vi "Front Panel.vi"(11 "GUI In":refnum<class "CRD Derived.lvclass">) -> ()   [LabVIEW 2015, in "CRD Derived.lvclass"]
uses:
  CRD Derived.lvclass
  Reusable/Xctls/Buffer/2D Control/2D Buffer Display.xctl
  Reusable/GUI/GUI.lvclass/GUI.ctl
  Reusable/Observer/Observer.lvclass/Observer.ctl
  CRDS/Data/cCRDS Data.lvclass
  Reusable/CRDS/Data/Cell/CRDS Cell Data.lvclass/CRDS Cell Data.ctl
  Reusable/CRDS/Data/Cell/Read extParam.vi
  Reusable/GUI/Accessors/Read RegEvent.vi
  Reusable/Observer/Read Data Queue.vi
  Reusable/CRDS/Data/Main/Read CellData.vi
  Reusable/Data/Read measTime.vi
  Reusable/Data/Data.lvclass
  Reusable/CRDS/Data/Cell/CRDS Cell Data.lvclass
panel:
  out "extWvfm":cluster{"data_out":sgl[][], "time":timestamp}(xcontrol)
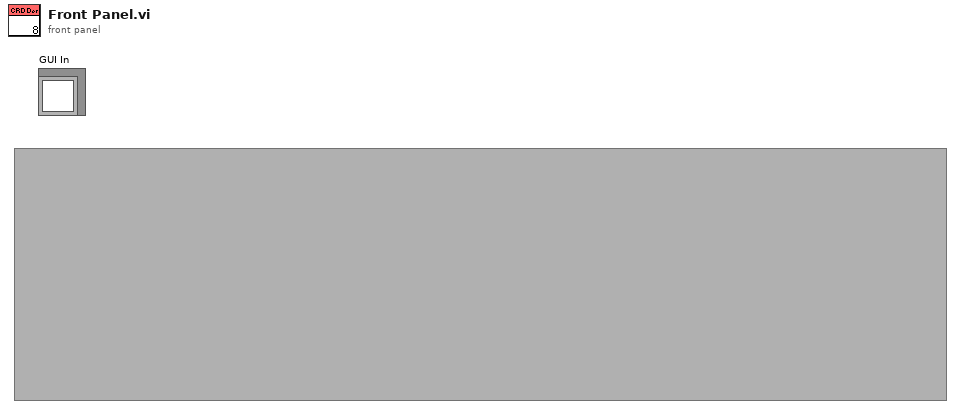
[diagram p1: front panel]
types:
  T1 = cluster{"Name":string, "Line Width":u8, "Line Style":u8, "Color":u32}[]
  T2 = typedef "extparam.ctl" = cluster{"Tau":sgl, "Tau0cor":sgl, "ext":sgl, "extCorr":sgl, "stdevTau":sgl, "eTau":sgl, "taucorr":sgl, "Tau0":sgl, "max":sgl}
  T3 = cluster{"Data Access:extParam":sgl[][], "Time":timestamp}
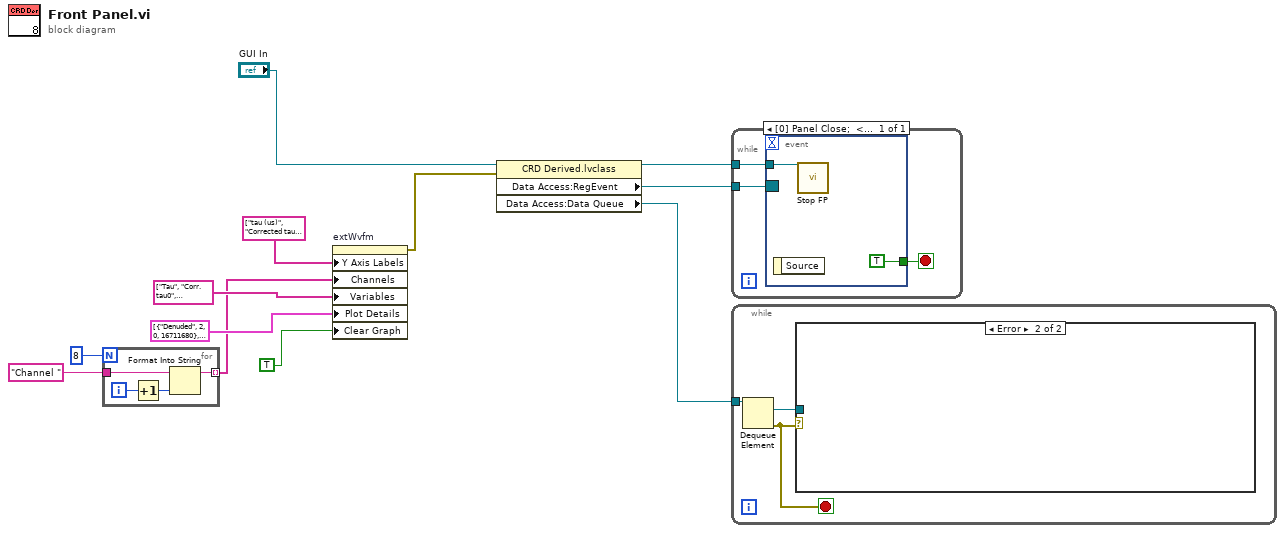
[diagram p0: block diagram]
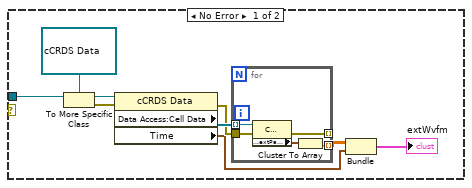
[diagram p2: hidden frame]
diagram:
  n1 = for {
    N: 8 -> [_]
    tunnel: "Channel " -> [w14]
    tunnel: [w13] -> w5 mode=indexing
    i -> [w16]
    n2 = Increment(x=w16) -> (x+1=w15:i32)
    n3 = Format Into String(initial string=w14, w15) -> (resulting string=w13:string)  [unwired: 2 in, 1 out]
  }
  n4 = property on="extWvfm" class="2D Buffer Display (strict)"("Y Axis Labels"=string[] ["tau (us)", "Corrected tau0 (us)", "Extinction (Mm-1)", "Corrected Extinction (Mm-1)", "Std. Dev. in tau (us)", "Error in tau", "Corrected tau (us)", "tau0 (us)", "Max Amplitude"], "Channels"=w5, "Variables"=string[] ["Tau", "Corr.  tau0", "Extinction", "Corrected Extinction", "Std. Dev. in tau", "Error in tau", "Corrected tau", "tau0", "Max Amplitude"], "Plot Details"=T1 [{"Name"="Denuded", "Line Width"=2, "Line Style"=0, "Color"=16711680}, {"Name"="Denuded", "Line Width"=2, "Line Style"=1, "Color"=16860}, {"Name"="Gas", "Line Width"=2, "Line Style"=0, "Color"=33023}, {"Name"="Dry", "Line Width"=2, "Line Style"=0, "Color"=16512}, {"Name"="Dry", "Line Width"=2, "Line Style"=0, "Color"=8388672}, {"Name"="Dry", "Line Width"=2, "Line Style"=1, "Color"=6618880}, {"Name"="Med RH", "Line Width"=2, "Line Style"=1, "Color"=1985280}, {"Name"="High RH", "Line Width"=2, "Line Style"=1, "Color"=32832}], "Clear Graph"=TRUE) -> (error out=w2:errorcluster)  [unwired: 2 in, 1 out]
  n5 = property class="CRD Derived.lvclass"(reference="GUI In", error in=w2) -> (reference out=w1:refnum<class "CRD Derived.lvclass">, "Data Access:RegEvent"=w12:refnum<event-registration>, "Data Access:Data Queue"=w11:refnum<queue>)  [unwired: 1 out]
  n6 = while {
    tunnel: w12 -> [w18]
    tunnel: w1 -> [w17]
    stop <- w19 stop-if-true
    n7 = event shown="[0] Panel Close;  <True>: User Event" {
      selector: w18 -> [_]
      dyn-events: _ -> [_]
      timeout: _ -> [_]
      tunnel: [TRUE] -> w19
      tunnel: w17 -> [w20]
      event Panel Close; User Event {
        n8 = event-data() -> ()  [unwired: 1 in, 1 out]
        n9 = call-dynamic "Stop FP.vi"("GUI in"=w20) -> ()  [unwired: 9 in, 2 out]
      }
    }
  }
  n10 = while {
    tunnel: w11 -> [w24]
    stop <- w23 stop-if-true
    n11 = Dequeue Element(queue=w24) -> (element=w22:refnum<data-value>, error out=w23:errorcluster)  [unwired: 2 in, 2 out]
    n12 = case shown="Error" w23 {
      tunnel: w22 -> [w31 _]
      frame No Error {
        n13 = To More Specific Class(target class=refnum<data-value> refnum ("data value reference"), reference=w31) -> (specific class reference=w30:refnum<data-value>, error out=w25:errorcluster)  [unwired: 1 in]
        n14 = property class="cCRDS Data"(reference=w30, error in=w25) -> (error out=w32:errorcluster, "Data Access:Cell Data"=w33:refnum<class "CRDS Cell Data.lvclass">[], "Time"=w27:timestamp)  [unwired: 1 out]
        n15 = for {
          tunnel: w33 -> [w38] mode=indexing
          tunnel: [w37] -> _ mode=indexing
          tunnel: w32 -> [w36]
          tunnel: [w34] -> w28 mode=indexing
          n16 = property class="CRDS Cell"(reference=w38, error in=w36) -> (error out=w37:errorcluster, "Data Access:extParam"=w35:T2)  [unwired: 1 out]
          n17 = Cluster To Array(cluster=w35) -> (array=w34:sgl[])
        }
        n18 = Bundle("Data Access:extParam"=w28, "Time"=w27) -> (→"extWvfm":T3)  [unwired: 1 in]
      }
      frame Error {
      }
    }
  }
